vi "Wait for Message.vi"(8 "error in":errorcluster, 10 "Timeout":i32 format="%d ms", 11 "epoll in":refnum<class "epoll.lvclass">) -> (0 "error out":errorcluster, 2 "Timed Out":bool, 3 "epoll out":refnum<class "epoll.lvclass">)   [LabVIEW 2018, in "PCANBasic.lvlib" / "epoll.lvclass"]
uses:
  epoll.lvclass
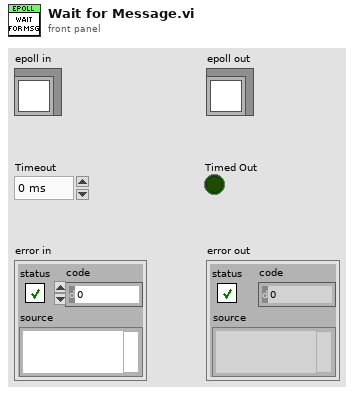
[diagram p1: front panel]
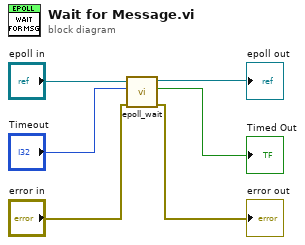
[diagram p0: block diagram]
diagram:
  n1 = call "epoll_wait.vi"("error in"="error in", "timeout ms"="Timeout", "epoll in"="epoll in") -> ("error out"=→"error out":errorcluster, "timed out"=→"Timed Out":bool, "epoll out"=→"epoll out":refnum<class "epoll.lvclass">)  [unwired: 6 in]
